vi "Enable Reference Output.vi"(0 "Mulde_board_settings_in":T1={"VISA resource name"="", "Address Space"=1, "window_offset"=0, "register_addresses"={"MM based Registers"={"Revision"=0, "OldestCompatRev"=0, "signature"=0, "scratch"=0, "LedControl"=0, "BoardHwRev"=0, "BoardControl"=0, "ThermalStatus"=0, "BasebandStatus"=0, "BasebandControl"=0, "BasebandAuxSetup"=0, "BasebandAuxStatus"=0, "LmkSyncOutSetup"=0, " AdcSyncOutSetup"=0, " InjSyncOutSetup"=0, " PxiTrig0OutSetup"=0, " PxiTrig1OutSetup"=0, " PxiTrig2OutSetup"=0, " PxiTrig3OutSetup"=0, " PxiTrig4OutSetup"=0, " PxiTrig5OutSetup"=0, " PxiTrig6OutSetup"=0, " PxiTrig7OutSetup"=0}, "CPLD based Registers"={"SlaveSignature"=0, "SlaveRevision"=0, "SlaveOldestCompatRev"=0, "SlaveScratch"=0, "SlaveSetup"=0, "SlaveStatus"=0, "IDacReg_offset"=0, "LMKRegGrp0_offset"=0, "QDacReg_offset"=0, "BrdTempSensorVal"=0, "TempSensorPowerDown"=0, "GPIOReg_offset"=0, "IAdcReg_offset"=0, "QAdcReg_offset"=0, "LMKRegGrp1_offset"=0, "QadcTempSensorVal"=0, "IadcTempSensorVal"=0, "RevisionReg"=0, "VcxoReg"=0, "CpldStatusReg"=0, "PowerReg"=0, "VBiasEnReg"=0, "ExtRefOeReg"=0, "QdacCtrlReg"=0, "QdacStatusReg"=0, "IdacCtrlReg"=0, "IdacStatusReg"=0, "QdacJtagIn"=0, "QdacJtagOut"=0, "IdacJtagIn"=0, "IdacJtagOut"=0, "IqDcSetupReg"=0, "QadcStatusReg"=0, "IadcStatusReg"=0, "BrdSetupReg"=0, "IqDcRevisionReg"=0, "PllStatusReg"=0, "EndpointScratchReg"=0, "AdcSyncCfgReg"=0, "IqCardOpampReg"=0}, "CPLD Register Offset"=0, "MM  Register Offset"=0, " PxiTrig0OutSetup"=0}, "required_MM_fpga_version"={"signature"=0, "hardware"=0, "current revision"=0, "oldest revision"=0}, "CPLD Oldest Compat Version "={"hardware"=0, "CPLD firmware"=0}, "MM_FPGA_image_location"="", "is_init"=FALSE, "card_type"=enum."ADC", "DacLmkConfigFileName"="", "AdcLmkConfigFileName"="", "AdcConfigFileName"="", "DacConfigFileName_RevA"="", "DacConfigFileName_RevB"="", "Mulde hardware revision"=0, "bypass DAC PLL\n"=FALSE, "IQ Card Revision"=enum."RevA", "board capability"={"baseband sync"=enum."no baseband sync"}} {"Address Space" items=["VXI/VME A16"=1, "VXI/VME A24"=2, "VXI/VME A32"=3, "VXI/VME A64"=4, "PXI Memory Allocations"=9, "PXI Configuration"=10, "PXI BAR0"=11, "PXI BAR1"=12, "PXI BAR2"=13, "PXI BAR3"=14, "PXI BAR4"=15, "PXI BAR5"=16]}, 5 "output reference enable":bool, 11 "error in":errorcluster) -> (4 "Mulde_board_settings_out":T1={"VISA resource name"="", "Address Space"=1, "window_offset"=0, "register_addresses"={"MM based Registers"={"Revision"=0, "OldestCompatRev"=0, "signature"=0, "scratch"=0, "LedControl"=0, "BoardHwRev"=0, "BoardControl"=0, "ThermalStatus"=0, "BasebandStatus"=0, "BasebandControl"=0, "BasebandAuxSetup"=0, "BasebandAuxStatus"=0, "LmkSyncOutSetup"=0, " AdcSyncOutSetup"=0, " InjSyncOutSetup"=0, " PxiTrig0OutSetup"=0, " PxiTrig1OutSetup"=0, " PxiTrig2OutSetup"=0, " PxiTrig3OutSetup"=0, " PxiTrig4OutSetup"=0, " PxiTrig5OutSetup"=0, " PxiTrig6OutSetup"=0, " PxiTrig7OutSetup"=0}, "CPLD based Registers"={"SlaveSignature"=0, "SlaveRevision"=0, "SlaveOldestCompatRev"=0, "SlaveScratch"=0, "SlaveSetup"=0, "SlaveStatus"=0, "IDacReg_offset"=0, "LMKRegGrp0_offset"=0, "QDacReg_offset"=0, "BrdTempSensorVal"=0, "TempSensorPowerDown"=0, "GPIOReg_offset"=0, "IAdcReg_offset"=0, "QAdcReg_offset"=0, "LMKRegGrp1_offset"=0, "QadcTempSensorVal"=0, "IadcTempSensorVal"=0, "RevisionReg"=0, "VcxoReg"=0, "CpldStatusReg"=0, "PowerReg"=0, "VBiasEnReg"=0, "ExtRefOeReg"=0, "QdacCtrlReg"=0, "QdacStatusReg"=0, "IdacCtrlReg"=0, "IdacStatusReg"=0, "QdacJtagIn"=0, "QdacJtagOut"=0, "IdacJtagIn"=0, "IdacJtagOut"=0, "IqDcSetupReg"=0, "QadcStatusReg"=0, "IadcStatusReg"=0, "BrdSetupReg"=0, "IqDcRevisionReg"=0, "PllStatusReg"=0, "EndpointScratchReg"=0, "AdcSyncCfgReg"=0, "IqCardOpampReg"=0}, "CPLD Register Offset"=0, "MM  Register Offset"=0, " PxiTrig0OutSetup"=0}, "required_MM_fpga_version"={"signature"=0, "hardware"=0, "current revision"=0, "oldest revision"=0}, "CPLD Oldest Compat Version "={"hardware"=0, "CPLD firmware"=0}, "MM_FPGA_image_location"="", "is_init"=FALSE, "card_type"=enum."ADC", "DacLmkConfigFileName"="", "AdcLmkConfigFileName"="", "AdcConfigFileName"="", "DacConfigFileName_RevA"="", "DacConfigFileName_RevB"="", "Mulde hardware revision"=0, "bypass DAC PLL\n"=FALSE, "IQ Card Revision"=enum."RevA", "board capability"={"baseband sync"=enum."no baseband sync"}} {"Address Space" items=["VXI/VME A16"=1, "VXI/VME A24"=2, "VXI/VME A32"=3, "VXI/VME A64"=4, "PXI Memory Allocations"=9, "PXI Configuration"=10, "PXI BAR0"=11, "PXI BAR1"=12, "PXI BAR2"=13, "PXI BAR3"=14, "PXI BAR4"=15, "PXI BAR5"=16]}, 15 "error out":errorcluster)   [LabVIEW 2019]
uses:
  <instrlib>/niMmWave/ni3610 and ni3630/controls/public/Main Settings.ctl
  <vilib>/Instr/_visa.llb/VISA Register Access Address Space.ctl
  <instrlib>/niMmWave/ni3610 and ni3630/controls/public/Register Adresses.ctl
  <instrlib>/niMmWave/ni3610 and ni3630/controls/public/Base Card Type.ctl
  <instrlib>/niMmWave/ni3610 and ni3630/controls/private/IQ Card Revision.ctl
  <instrlib>/niMmWave/ni3610 and ni3630/controls/public/Board Capability.ctl
  <instrlib>/niMmWave/ni3610 and ni3630/ni3610_and_ni3630_Driver_Lib.lvlib
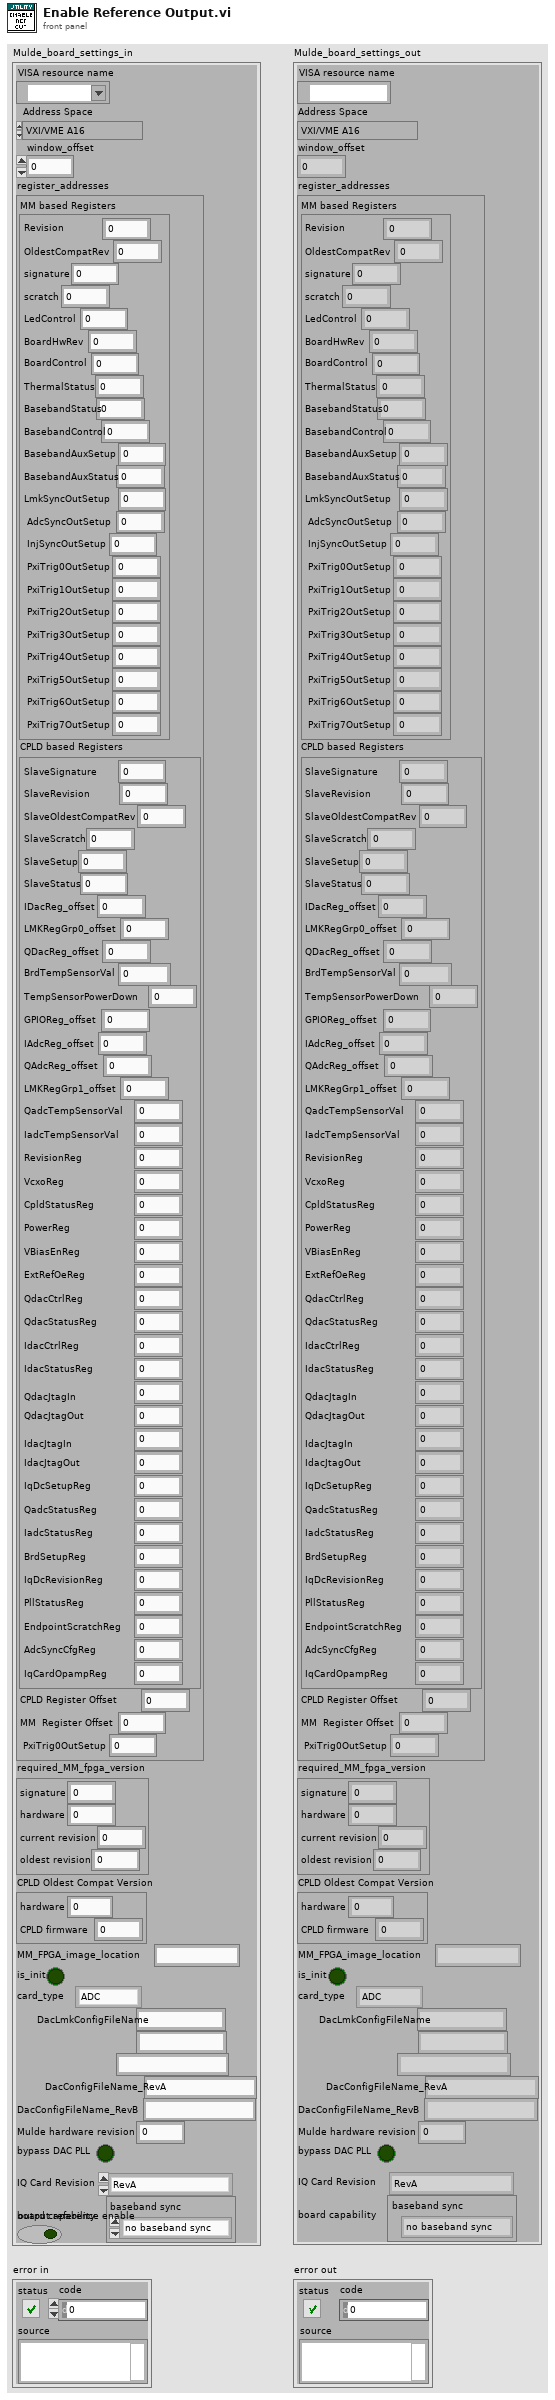
[diagram p1: front panel]
types:
  T1 = typedef "ni3610_and_ni3630_Driver_Lib.lvlib/Main Settings.ctl" = cluster{"VISA resource name":refnum<visa-resource-name>, "Address Space":T2, "window_offset":u32, "register_addresses":T3, "required_MM_fpga_version":cluster{"signature":u32, "hardware":u32, "current revision":u32, "oldest revision":u32}, "CPLD Oldest Compat Version ":cluster{"hardware":u32, "CPLD firmware":u32}, "MM_FPGA_image_location":string, "is_init":bool, "card_type":T4, "DacLmkConfigFileName":string, "AdcLmkConfigFileName":string, "AdcConfigFileName":string, "DacConfigFileName_RevA":string, "DacConfigFileName_RevB":string, "Mulde hardware revision":u8, "bypass DAC PLL\n":bool, "IQ Card Revision":T5, "board capability":T6}
  T2 = typedef "VISA Register Access Address Space.ctl" = u16
  T3 = typedef "ni3610_and_ni3630_Driver_Lib.lvlib/Register Adresses.ctl" = cluster{"MM based Registers":cluster{"Revision":u32, "OldestCompatRev":u32, "signature":u32, "scratch":u32, "LedControl":u32, "BoardHwRev":u32, "BoardControl":u32, "ThermalStatus":u32, "BasebandStatus":u32, "BasebandControl":u32, "BasebandAuxSetup":u32, "BasebandAuxStatus":u32, "LmkSyncOutSetup":u32, " AdcSyncOutSetup":u32, " InjSyncOutSetup":u32, " PxiTrig0OutSetup":u32, " PxiTrig1OutSetup":u32, " PxiTrig2OutSetup":u32, " PxiTrig3OutSetup":u32, " PxiTrig4OutSetup":u32, " PxiTrig5OutSetup":u32, " PxiTrig6OutSetup":u32, " PxiTrig7OutSetup":u32}, "CPLD based Registers":cluster{"SlaveSignature":u32, "SlaveRevision":u32, "SlaveOldestCompatRev":u32, "SlaveScratch":u32, "SlaveSetup":u32, "SlaveStatus":u32, "IDacReg_offset":u32, "LMKRegGrp0_offset":u32, "QDacReg_offset":u32, "BrdTempSensorVal":u32, "TempSensorPowerDown":u32, "GPIOReg_offset":u32, "IAdcReg_offset":u32, "QAdcReg_offset":u32, "LMKRegGrp1_offset":u32, "QadcTempSensorVal":u32, "IadcTempSensorVal":u32, "RevisionReg":u32, "VcxoReg":u32, "CpldStatusReg":u32, "PowerReg":u32, "VBiasEnReg":u32, "ExtRefOeReg":u32, "QdacCtrlReg":u32, "QdacStatusReg":u32, "IdacCtrlReg":u32, "IdacStatusReg":u32, "QdacJtagIn":u32, "QdacJtagOut":u32, "IdacJtagIn":u32, "IdacJtagOut":u32, "IqDcSetupReg":u32, "QadcStatusReg":u32, "IadcStatusReg":u32, "BrdSetupReg":u32, "IqDcRevisionReg":u32, "PllStatusReg":u32, "EndpointScratchReg":u32, "AdcSyncCfgReg":u32, "IqCardOpampReg":u32}, "CPLD Register Offset":u32, "MM  Register Offset":u32, " PxiTrig0OutSetup":u32}
  T4 = typedef "ni3610_and_ni3630_Driver_Lib.lvlib/Base Card Type.ctl" = enum16{"unspecified", "ADC", "DAC"}
  T5 = typedef "ni3610_and_ni3630_Driver_Lib.lvlib/IQ Card Revision.ctl" = enum16{"RevA", "RevB", "RevC", "RevD"}
  T6 = typedef "ni3610_and_ni3630_Driver_Lib.lvlib/Board Capability.ctl" = cluster{"baseband sync":enum16{"no baseband sync", "baseband sync"}}
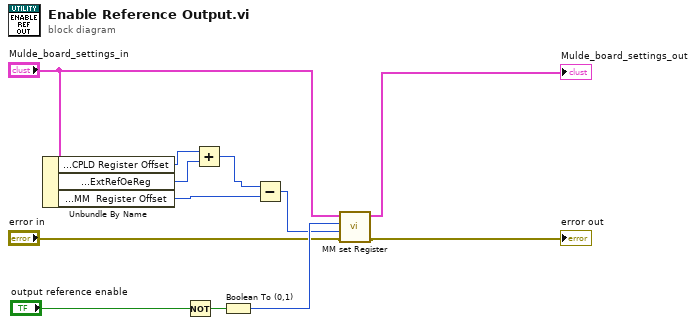
[diagram p0: block diagram]
diagram:
  n1 = Unbundle By Name("Mulde_board_settings_in") -> ("register_addresses.CPLD Register Offset"=w5:u32, "register_addresses.CPLD based Registers.ExtRefOeReg"=w4:u32, "register_addresses.MM  Register Offset"=w3:u32)
  n2 = Not(x="output reference enable") -> (.not. x?=w11:bool)
  n3 = Add(x=w5, y=w4) -> (x+y=w2:u32)
  n4 = Boolean To (0,1)(Boolean=w11) -> (0, 1=w8:i16)
  n5 = Subtract(x=w2, y=w3) -> (x-y=w1:u32)
  n6 = call <instrlib>:"MM set Register.vi"("error in"="error in", "MM address"=w1, "Value"=w8, "Board Settings in"="Mulde_board_settings_in") -> ("error out"=→"error out":errorcluster, "Board Settings out"=→"Mulde_board_settings_out":T1)  [unwired: 6 in]
